vi "Return Activate Status.vi"(6 "error":string, 8 "error in (no error)":errorcluster, 9 "Status":T1, 11 "SCADA in":refnum<class "SCADA.lvclass">) -> (0 "error out":errorcluster, 3 "SCADA out":refnum<class "SCADA.lvclass">)   [LabVIEW 2015, in "SCADA Core.lvlib" / "SCADA.lvclass"]
uses:
  SCADA.lvclass
  SCADA Abstract Messages/Simple Command Status Msg/Simple Command Status.ctl
  SCADA.lvclass/SCADA.ctl
  <vilib>/ActorFramework/Actor/Actor.lvclass/Actor.ctl
  Controls/Grid Mode.ctl
  <vilib>/ActorFramework/Actor/Actor.lvclass
  SCADA Abstract Messages/Simple Command Status Msg/Simple Command Status Msg.lvclass
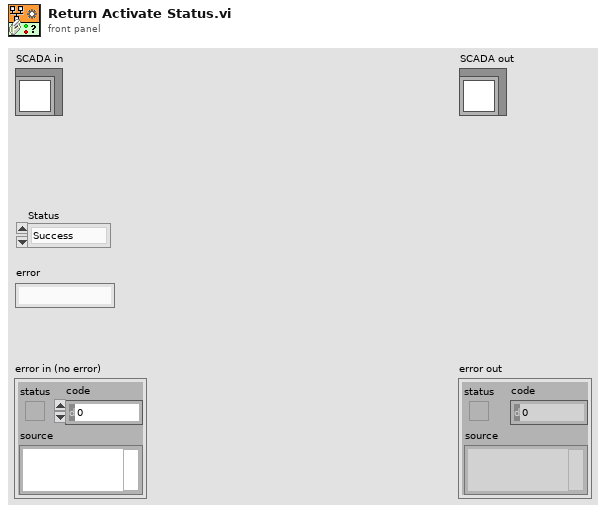
[diagram p1: front panel]
types:
  T1 = typedef "SCADA Core.lvlib/Simple Command Status Msg.lvclass/Simple Command Status.ctl" = enum16{"Success", "Failure"}
  T2 = typedef "SCADA Core.lvlib/SCADA.lvclass/Grid Mode.ctl" = enum16{"Off", "Grid Connected", "Islanded", "Synchronizing"}
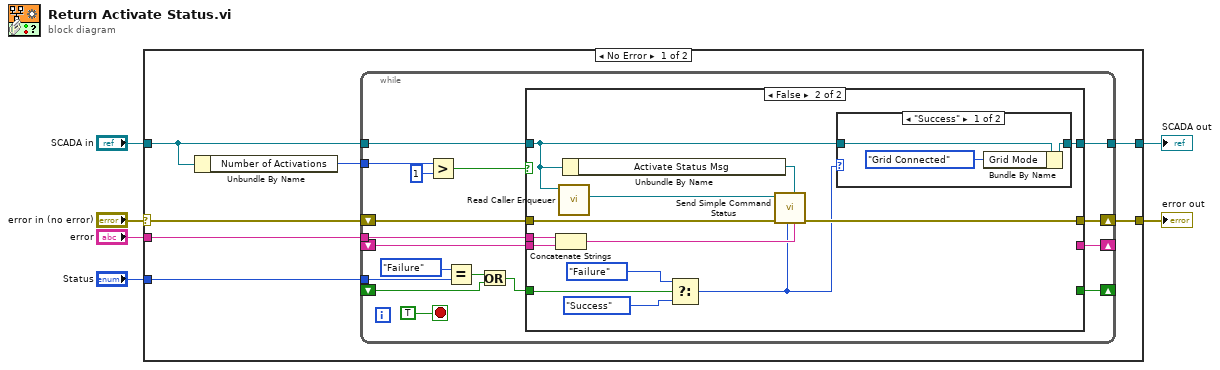
[diagram p0: block diagram]
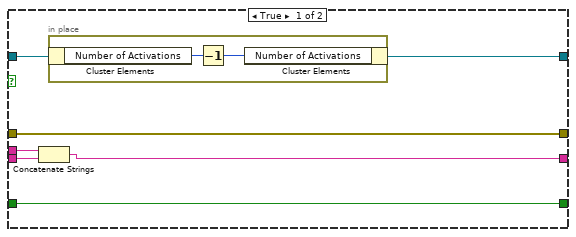
[diagram p2: hidden frame]
diagram:
  n1 = case shown="No Error" "error in (no error)" {
    selector: "error in (no error)" -> [w13 w58]
    tunnel: [w12 w58] -> w2
    tunnel: [w8 w57] -> w1
    tunnel: "SCADA in" -> [w9 w57]
    tunnel: "error" -> [w11 _]
    tunnel: "Status" -> [w10 _]
    frame No Error {
      n2 = Unbundle By Name(w9) -> ("Number of Activations"=w7:i32)
      n3 = while {
        tunnel: w9 -> [w19]
        tunnel: w11 -> [w23]
        tunnel: w10 -> [w25]
        shift-right: [w29] -> _
        shift-left: _ -> [w26]
        shift-right: [w22] -> _
        shift-left: _ -> [w21]
        shift-right: [w18] -> w12
        shift-left: w13 -> [w20]
        tunnel: [w17] -> w8
        tunnel: w7 -> [w15]
        stop <- TRUE stop-if-true
        n4 = Greater?(x=w15, y=1) -> (0:w14:bool)
        n5 = Equal?(x=Simple_Command_Status."Failure" ("y"), y=w25) -> (x = y?=w28:bool)
        n6 = Or(x=w28, y=w26) -> (x .or. y?=w24:bool)
        n7 = case shown="False" w14 {
          tunnel: [w37 _] -> w29
          tunnel: w24 -> [w37 w50]
          tunnel: w23 -> [w36 w52]
          tunnel: [w35 _] -> w22
          tunnel: w21 -> [w34 w51]
          tunnel: w20 -> [w33 w45]
          tunnel: w19 -> [w32 w42]
          tunnel: [w33 w43] -> w18
          tunnel: [w31 w41] -> w17
          frame True {
            n8 = Concatenate Strings(w36, w34) -> (w35:string)
            n9 = in-place {
              n10 = in-place-cluster #1(w32) -> ("Number of Activations"=w39:i32)
              n11 = Decrement(x=w39) -> (x-1=w38:i32)
              n12 = in-place-cluster #1("Number of Activations"=w38) -> (w31:refnum<class "SCADA.lvclass">)
            }
          }
          frame False {
            n13 = Concatenate Strings(w52, w51) -> (w44:string)
            n14 = call <vilib>:"Read Caller Enqueuer.vi"("Actor"=w42) -> ("Caller Enqueuer"=w46:refnum<class "Message Enqueuer.lvclass">)  [unwired: 10 in]
            n15 = Unbundle By Name(w42) -> ("Activate Status Msg"=w47:refnum<class "Simple Command Status Msg.lvclass">)
            n16 = Select(t=Simple_Command_Status."Failure" ("y"), s=w50, f=Simple_Command_Status."Success" ("y")) -> (s? t:f=w40:T1)
            n17 = call "Send Simple Command Status.vi"("error"=w44, "Simple Command Status Msg"=w47, "Status"=w40, "error in (no error)"=w45, "Message Enqueuer in"=w46) -> ("error out"=w43:errorcluster)  [unwired: 5 in, 1 out]
            n18 = case shown="\"Success\"" w40 {
              tunnel: w42 -> [w55 w56]
              tunnel: [w54 w56] -> w41
              frame "Success" {
                n19 = Bundle By Name(cluster=w55, "Grid Mode"=Grid_Mode."Grid Connected") -> (w54:refnum<class "SCADA.lvclass">)
              }
              frame "Failure" {
              }
            }
          }
        }
      }
    }
    frame Error {
    }
  }
  "error out" <- w2
  "SCADA out" <- w1
